vi "Write Graph_Ref.vi"(8 "error in":errorcluster, 10 "Graph_Ref":refnum<vi>, 11 "Report Viewer in":refnum<class "Report Viewer.lvclass">) -> (0 "error out":errorcluster, 3 "Report Viewer out":refnum<class "Report Viewer.lvclass">)   [LabVIEW 2023, in "Report Viewer.lvlib" / "Report Viewer.lvclass"]
uses:
  Library/Report Viewer.lvclass
  Library/Report Viewer.lvclass/Report Viewer.ctl
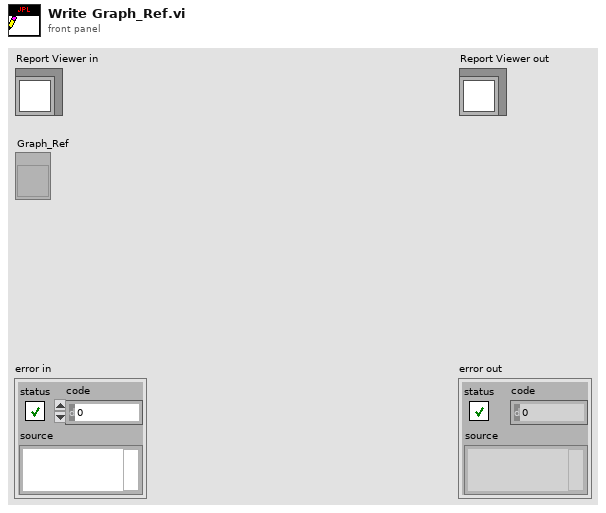
[diagram p1: front panel]
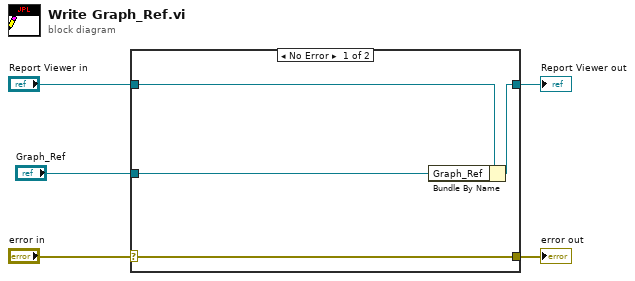
[diagram p0: block diagram]
diagram:
  n1 = case shown="No Error" "error in" {
    selector: "error in" -> [w9 w10]
    tunnel: [w9 w10] -> w4
    tunnel: [w7 w11] -> w2
    tunnel: "Report Viewer in" -> [w8 w11]
    tunnel: "Graph_Ref" -> [w6 _]
    frame No Error {
      n2 = Bundle By Name(cluster=w8, "Graph_Ref"=w6) -> (w7:refnum<class "Report Viewer.lvclass">)
    }
    frame Error {
    }
  }
  "error out" <- w4
  "Report Viewer out" <- w2
